vi "Configure.vi"(8 "error in (no error)":errorcluster, 11 "Function in":refnum<class "Function.lvclass">) -> (0 "error out":errorcluster, 3 "Function out":refnum<class "Function.lvclass">)   [LabVIEW 2016, in "Function Actor.lvlib" / "Function.lvclass"]
doc: "Override configure.vi to setup any parameters for a function before acquiring.\n\nConfigure.vi is called by the 'Initialize Function Actor Core.vi,' which executes before Actor Core of the root function class. The root configure method populates the basic Function UI with information such as the hardware device in use and the name of the function. The base configure method calls 'Acquire.vi' once execution is complete. If beginning a recurring acquisition, it reset the iteration count to zero."
uses:
  <userlib>/Common Components/Function Actor/Function.lvclass
  <userlib>/Common Components/Function Actor/Function.lvclass/Function.ctl
  <userlib>/Common Components/Slave Configuration/Slave Config.lvclass
  <userlib>/Common Components/Slave Configuration/Slave Config.lvclass/Slave Config.ctl
  <userlib>/Common Components/Slave Configuration/Config/Read IP Address of Server.vi
  <userlib>/Common Components/Slave Configuration/Config/Read remote port.vi
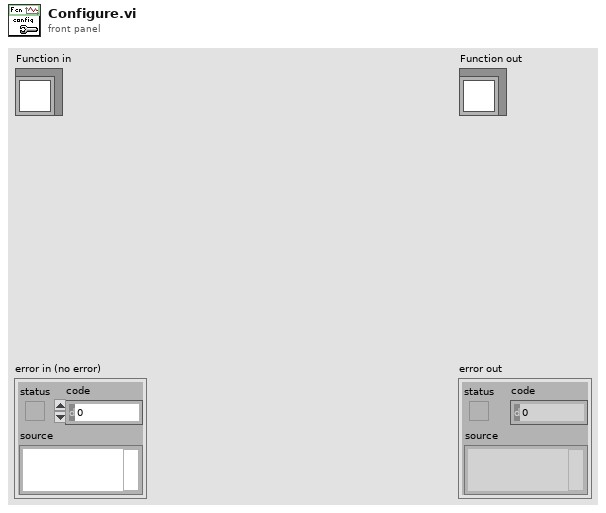
[diagram p1: front panel]
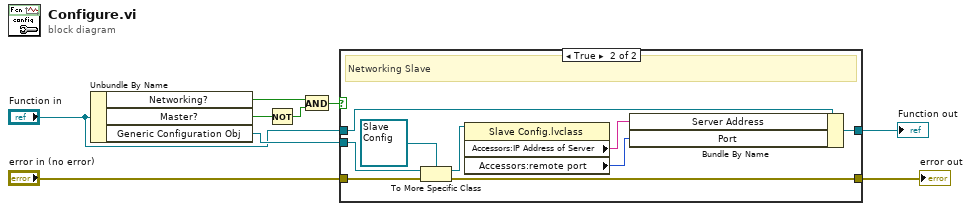
[diagram p0: block diagram]
diagram:
  n1 = Unbundle By Name("Function in") -> ("Networking?"=w9:bool, "Master?"=w8:bool, "Generic Configuration Obj"=w5:refnum<class "Configuration.lvclass">)
  n2 = Not(x=w8) -> (.not. x?=w7:bool)
  n3 = And(x=w9, y=w7) -> (x .and. y?=w6:bool)
  n4 = case shown="True" w6 {
    tunnel: w5 -> [_ w20]
    tunnel: "error in (no error)" -> [w10 w19]
    tunnel: "Function in" -> [w11 w16]
    tunnel: [w11 w13] -> w2
    tunnel: [w10 w12] -> w1
    frame False {
    }
    frame True {
      # "Networking Slave"
      n5 = To More Specific Class(target class=refnum<class "Slave Config.lvclass"> refnum ("Slave Config.lvclass"), reference=w20, error in=w19) -> (specific class reference=w17:refnum<class "Slave Config.lvclass">, error out=w12:errorcluster)
      n6 = property class="Slave Config.lvclass"(reference=w17) -> ("Accessors:IP Address of Server"=w15:string, "Accessors:remote port"=w14:u16)  [unwired: 1 in, 2 out]
      n7 = Bundle By Name(cluster=w16, "Server Address"=w15, "Port"=w14) -> (w13:refnum<class "Function.lvclass">)
    }
  }
  "error out" <- w1
  "Function out" <- w2
